vi "TresholdToTheta.vi"(2 "Treshold [dB]":dbl format="%#_13g", 3 "Power Max [W]":dbl format="%#_13g", 4 "Power now [W]":dbl format="%#_13g") -> (0 "Direction":i32, 1 "theta":dbl format="%#_13g")   [LabVIEW 2018]
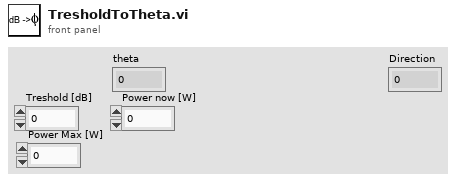
[diagram p1: front panel]
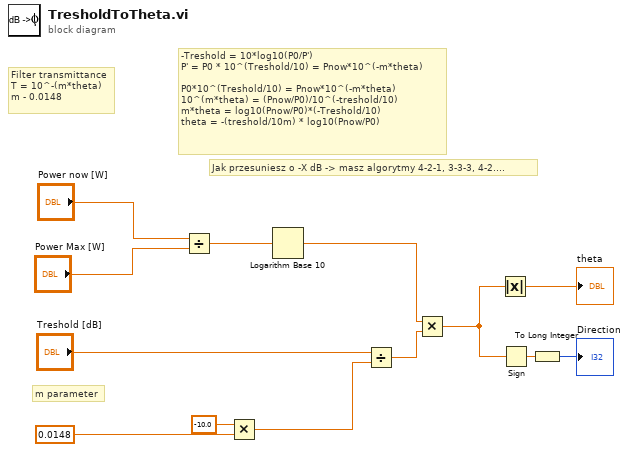
[diagram p0: block diagram]
diagram:
  # "Jak przesuniesz o -X dB -> masz algorytmy 4-2-1, 3-3-3, 4-2...."
  # "-Treshold = 10*log10(P0/P')\nP' = P0 * 10^(Treshold/10) = Pnow*10^(-m*theta)\n\nP0*10^(Treshold/10) = Pnow*10^(-m*theta)\n10^(m*theta) = (Pnow/P0)/10^(-treshold/10)\nm*theta = log10(Pnow/P0)*(-Treshold/10)\ntheta = -(treshold/10m) * log10(Pnow/P0)"
  # "m parameter"
  # "Filter transmittance\nT = 10^-(m*theta)\nm - 0.0148"
  n1 = Divide(x="Power now [W]", y="Power Max [W]") -> (x/y=w4:dbl)
  n2 = Multiply(x=-10.0, y=0.0148) -> (x*y=w8:dbl)
  n3 = Logarithm Base 10(1:w4) -> (0:w2:dbl)
  n4 = Divide(x="Treshold [dB]", y=w8) -> (x/y=w3:dbl)
  n5 = Multiply(x=w2, y=w3) -> (x*y=w1:dbl)
  n6 = Absolute Value(x=w1) -> (abs(x)=→"theta":dbl)
  n7 = Sign(1:w1) -> (0:w12:dbl)
  n8 = To Long Integer(number=w12) -> (32bit integer=→"Direction":i32)
